vi "error handler.vi"(8 "error in (no error)":errorcluster, 10 "JSON of invalid tags (optional)":string, 11 "Success Message":string) -> (0 "error out":errorcluster, 2 "Response String":string, 3 "Response Code":i32)   [LabVIEW 2013]
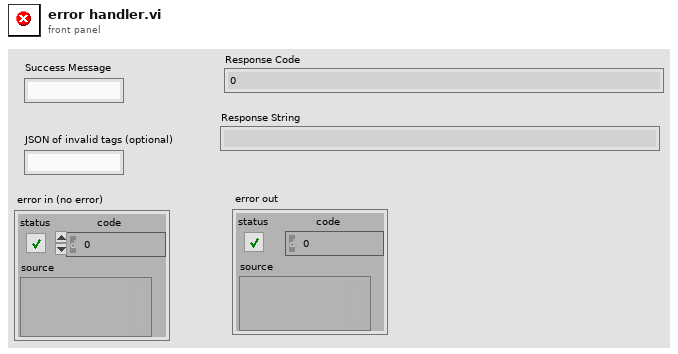
[diagram p1: front panel]
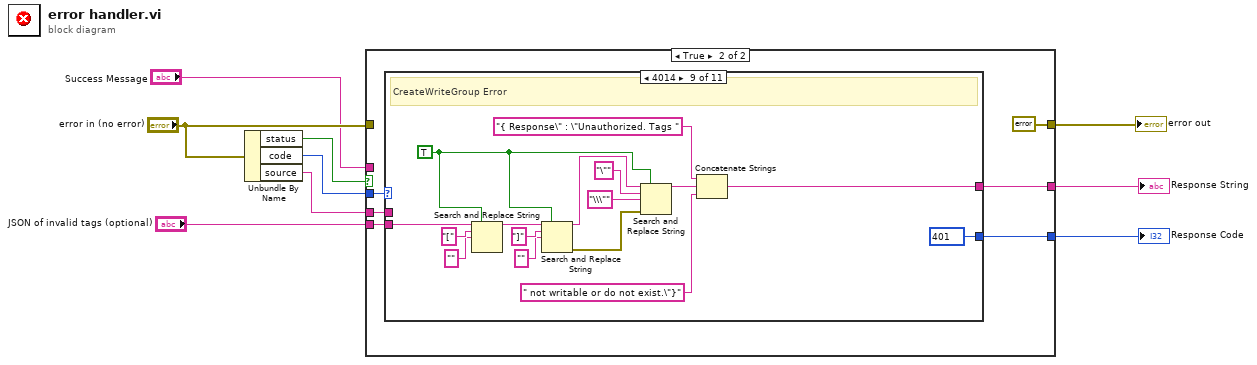
[diagram p0: block diagram]
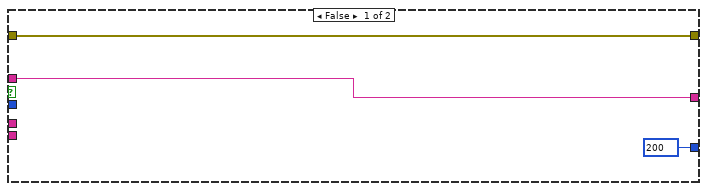
[diagram p2: hidden frame]
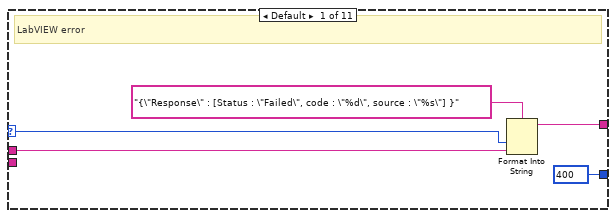
[diagram p3: hidden frame]
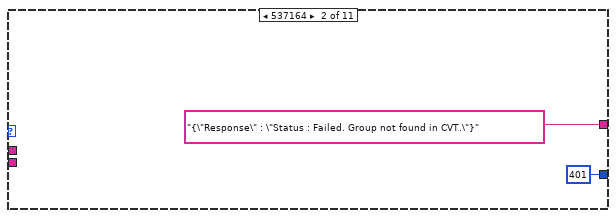
[diagram p4: hidden frame]
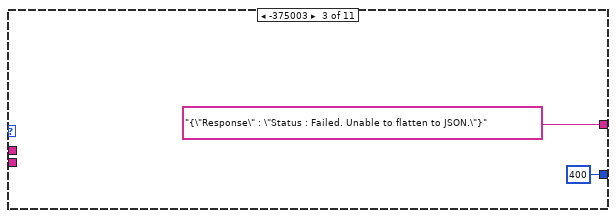
[diagram p5: hidden frame]
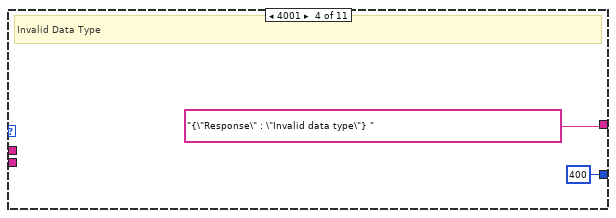
[diagram p6: hidden frame]
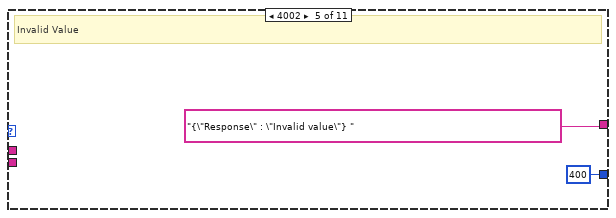
[diagram p7: hidden frame]
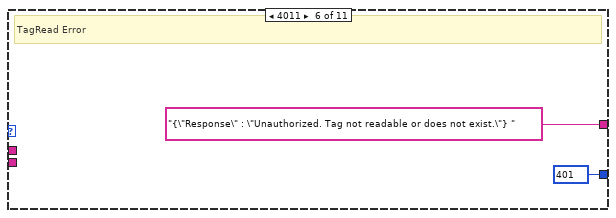
[diagram p8: hidden frame]
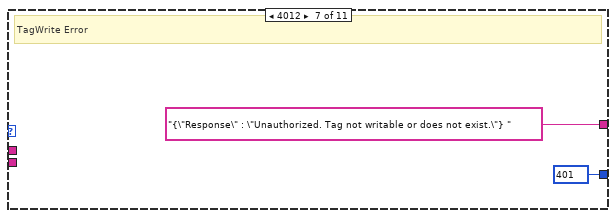
[diagram p9: hidden frame]
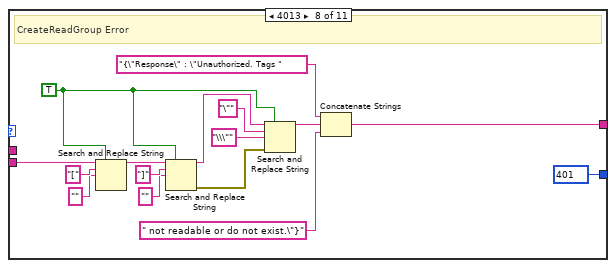
[diagram p10: hidden frame]
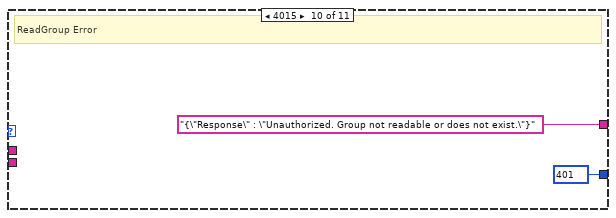
[diagram p11: hidden frame]
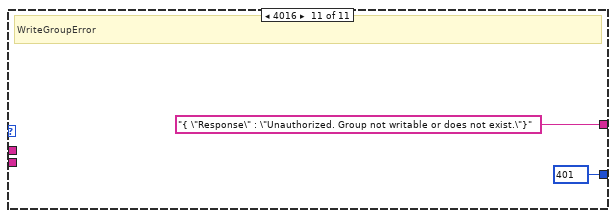
[diagram p12: hidden frame]
diagram:
  n1 = Unbundle By Name("error in (no error)") -> ("status"=w7:bool, "code"=w9:i32, "source"=w8:string)
  n2 = case shown="True" w7 {
    tunnel: w9 -> [_ w18]
    tunnel: w8 -> [_ w17]
    tunnel: "JSON of invalid tags (optional)" -> [_ w16]
    tunnel: [w12 w15] -> w6
    tunnel: [w11 errorcluster {"status"=FALSE, "code"=0, "source"=""} ("error in (no error)")] -> w5
    tunnel: "error in (no error)" -> [w11 _]
    tunnel: "Success Message" -> [w10 _]
    tunnel: [w10 w13] -> w2
    frame False {
      w12 = 200 items=["100"=100, "101"=101, "200"=200, "201"=201, "202"=202, "203"=203, "204"=204, "205"=205, "206"=206, "300"=300, "301"=301, "302"=302, "303"=303, "304"=304, "305"=305, "306"=306, "307"=307, "400"=400, "401"=401, "402"=402, "403"=403, "404"=404, "405"=405, "406"=406, "407"=407, "408"=408, "409"=409, "410"=410, "411"=411, "412"=412, "413"=413, "414"=414, "415"=415, "416"=416, "417"=417, "500"=500, "501"=501, "502"=502, "503"=503, "504"=504, "505"=505] ("response code (200)")
    }
    frame True {
      n3 = case shown="4014" w18 {
        selector: w18 -> [w21 _ _ _ _ _ _ _ _ _ _]
        tunnel: w17 -> [w20 _ _ _ _ _ _ _ _ _ _]
        tunnel: [w23 401 ("response code (200)") 400 ("response code (200)") 400 ("response code (200)") 400 ("response code (200)") w33 w35 w51 w67 w69 w71] -> w15
        tunnel: [w19 "{\"Response\" : \"Status : Failed. Group not found in CVT.\"}" ("format string") "{\"Response\" : \"Status : Failed. Unable to flatten to JSON.\"}" ("format string") "{\"Response\" : \"Invalid data type\"} " ("format string") "{\"Response\" : \"Invalid value\"} " ("format string") "{\"Response\" : \"Unauthorized. Tag not readable or does not exist.\"} " ("format string") "{\"Response\" : \"Unauthorized. Tag not writable or does not exist.\"} " ("format string") w36 w52 "{\"Response\" : \"Unauthorized. Group not readable or does not exist.\"}" ("format string") "{ \"Response\" : \"Unauthorized. Group not writable or does not exist.\"}" ("format string")] -> w13
        tunnel: w16 -> [_ _ _ _ _ _ _ w38 w54 _ _]
        frame Default {
          w23 = 400 items=["100"=100, "101"=101, "200"=200, "201"=201, "202"=202, "203"=203, "204"=204, "205"=205, "206"=206, "300"=300, "301"=301, "302"=302, "303"=303, "304"=304, "305"=305, "306"=306, "307"=307, "400"=400, "401"=401, "402"=402, "403"=403, "404"=404, "405"=405, "406"=406, "407"=407, "408"=408, "409"=409, "410"=410, "411"=411, "412"=412, "413"=413, "414"=414, "415"=415, "416"=416, "417"=417, "500"=500, "501"=501, "502"=502, "503"=503, "504"=504, "505"=505] ("response code (200)")
          # "LabVIEW error"
          n4 = Format Into String(format string="{\"Response\" : [Status : \"Failed\", code : \"%d\", source : \"%s\"] }", w21, w20) -> (resulting string=w19:string)  [unwired: 2 in, 1 out]
        }
        frame 537164 {
        }
        frame -375003 {
        }
        frame 4001 {
          # "Invalid Data Type"
        }
        frame 4002 {
          # "Invalid Value"
        }
        frame 4011 {
          w33 = 401 items=["100"=100, "101"=101, "200"=200, "201"=201, "202"=202, "203"=203, "204"=204, "205"=205, "206"=206, "300"=300, "301"=301, "302"=302, "303"=303, "304"=304, "305"=305, "306"=306, "307"=307, "400"=400, "401"=401, "402"=402, "403"=403, "404"=404, "405"=405, "406"=406, "407"=407, "408"=408, "409"=409, "410"=410, "411"=411, "412"=412, "413"=413, "414"=414, "415"=415, "416"=416, "417"=417, "500"=500, "501"=501, "502"=502, "503"=503, "504"=504, "505"=505] ("response code (200)")
          # "TagRead Error"
        }
        frame 4012 {
          w35 = 401 items=["100"=100, "101"=101, "200"=200, "201"=201, "202"=202, "203"=203, "204"=204, "205"=205, "206"=206, "300"=300, "301"=301, "302"=302, "303"=303, "304"=304, "305"=305, "306"=306, "307"=307, "400"=400, "401"=401, "402"=402, "403"=403, "404"=404, "405"=405, "406"=406, "407"=407, "408"=408, "409"=409, "410"=410, "411"=411, "412"=412, "413"=413, "414"=414, "415"=415, "416"=416, "417"=417, "500"=500, "501"=501, "502"=502, "503"=503, "504"=504, "505"=505] ("response code (200)")
          # "TagWrite Error"
        }
        frame 4013 {
          w39 = TRUE ("replace all? (F)")
          w51 = 401 items=["100"=100, "101"=101, "200"=200, "201"=201, "202"=202, "203"=203, "204"=204, "205"=205, "206"=206, "300"=300, "301"=301, "302"=302, "303"=303, "304"=304, "305"=305, "306"=306, "307"=307, "400"=400, "401"=401, "402"=402, "403"=403, "404"=404, "405"=405, "406"=406, "407"=407, "408"=408, "409"=409, "410"=410, "411"=411, "412"=412, "413"=413, "414"=414, "415"=415, "416"=416, "417"=417, "500"=500, "501"=501, "502"=502, "503"=503, "504"=504, "505"=505] ("response code (200)")
          # "CreateReadGroup Error"
          n5 = Search and Replace String(replace all?=w39, input string=w38, search string="[", replace string="" ("replace string (\"\")")) -> (result string=w46:string)  [unwired: 4 in, 3 out]
          n6 = Search and Replace String(replace all?=w39, input string=w46, search string="]", replace string="" ("replace string (\"\")")) -> (result string=w43:string, error out=w42:errorcluster)  [unwired: 4 in, 2 out]
          n7 = Search and Replace String(replace all?=w39, input string=w43, search string="\"", replace string="\\\"" ("replace string (\"\")"), error in=w42) -> (result string=w37:string)  [unwired: 3 in, 3 out]
          n8 = Concatenate Strings("{\"Response\" : \"Unauthorized. Tags " ("string"), w37, " not readable or do not exist.\"}" ("string")) -> (w36:string)
        }
        frame 4014 {
          w55 = TRUE ("replace all? (F)")
          w67 = 401 items=["100"=100, "101"=101, "200"=200, "201"=201, "202"=202, "203"=203, "204"=204, "205"=205, "206"=206, "300"=300, "301"=301, "302"=302, "303"=303, "304"=304, "305"=305, "306"=306, "307"=307, "400"=400, "401"=401, "402"=402, "403"=403, "404"=404, "405"=405, "406"=406, "407"=407, "408"=408, "409"=409, "410"=410, "411"=411, "412"=412, "413"=413, "414"=414, "415"=415, "416"=416, "417"=417, "500"=500, "501"=501, "502"=502, "503"=503, "504"=504, "505"=505] ("response code (200)")
          # "CreateWriteGroup Error"
          n9 = Search and Replace String(replace all?=w55, input string=w54, search string="[", replace string="" ("replace string (\"\")")) -> (result string=w62:string)  [unwired: 4 in, 3 out]
          n10 = Search and Replace String(replace all?=w55, input string=w62, search string="]", replace string="" ("replace string (\"\")")) -> (result string=w59:string, error out=w58:errorcluster)  [unwired: 4 in, 2 out]
          n11 = Search and Replace String(replace all?=w55, input string=w59, search string="\"", replace string="\\\"" ("replace string (\"\")"), error in=w58) -> (result string=w53:string)  [unwired: 3 in, 3 out]
          n12 = Concatenate Strings("{ Response\" : \"Unauthorized. Tags " ("string"), w53, " not writable or do not exist.\"}" ("string")) -> (w52:string)
        }
        frame 4015 {
          w69 = 401 items=["100"=100, "101"=101, "200"=200, "201"=201, "202"=202, "203"=203, "204"=204, "205"=205, "206"=206, "300"=300, "301"=301, "302"=302, "303"=303, "304"=304, "305"=305, "306"=306, "307"=307, "400"=400, "401"=401, "402"=402, "403"=403, "404"=404, "405"=405, "406"=406, "407"=407, "408"=408, "409"=409, "410"=410, "411"=411, "412"=412, "413"=413, "414"=414, "415"=415, "416"=416, "417"=417, "500"=500, "501"=501, "502"=502, "503"=503, "504"=504, "505"=505] ("response code (200)")
          # "ReadGroup Error"
        }
        frame 4016 {
          w71 = 401 items=["100"=100, "101"=101, "200"=200, "201"=201, "202"=202, "203"=203, "204"=204, "205"=205, "206"=206, "300"=300, "301"=301, "302"=302, "303"=303, "304"=304, "305"=305, "306"=306, "307"=307, "400"=400, "401"=401, "402"=402, "403"=403, "404"=404, "405"=405, "406"=406, "407"=407, "408"=408, "409"=409, "410"=410, "411"=411, "412"=412, "413"=413, "414"=414, "415"=415, "416"=416, "417"=417, "500"=500, "501"=501, "502"=502, "503"=503, "504"=504, "505"=505] ("response code (200)")
          # "WriteGroupError"
        }
      }
    }
  }
  "error out" <- w5
  "Response Code" <- w6
  "Response String" <- w2
